vi "Asset To UID.vi"(11 "Asset":T1) -> (3 "UID":i32)   [LabVIEW 2019]
doc: "Convert the enum to the corresponding UID found on the block diagram of BD Graphics.vi"
uses:
  Asset Enum.ctl
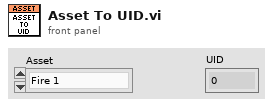
[diagram p1: front panel]
types:
  T1 = typedef "Asset Enum.ctl" = enum16{"Fire 1", "Fire 2", "Rubble"}
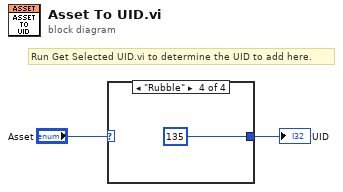
[diagram p0: block diagram]
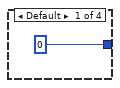
[diagram p2: hidden frame]
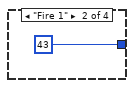
[diagram p3: hidden frame]
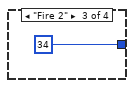
[diagram p4: hidden frame]
diagram:
  # "Run Get Selected UID.vi to determine the UID to add here."
  n1 = case shown="\"Rubble\"" "Asset" {
    tunnel: [0 43 34 135] -> w1
    frame Default {
    }
    frame "Fire 1" {
    }
    frame "Fire 2" {
    }
    frame "Rubble" {
    }
  }
  "UID" <- w1
